vi "Eval y=f(a,x1,x2) Prep.vi"(0 "Variables":string[](array[string]), 1 "formula":string, 2 "Parameters":cluster{string, dbl}[](array[cluster]) {"?" format="%.2f"}, 3 "Start":dbl[](array[numeric]) format="%.2f", 5 "End":dbl[](array[numeric]) format="%.2f") -> (4 "error situation 2":bool, 6 "formula copy":string, 7 "time [msec]":u32, 8 "error situation 1":bool, 9 "error (general)":bool)   [LabVIEW 2017, in "NI_Gmath.lvlib"]
uses:
  NI_Gmath.lvlib
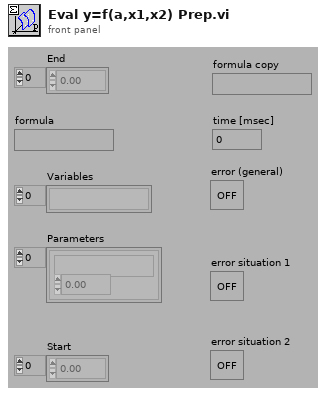
[diagram p1: front panel]
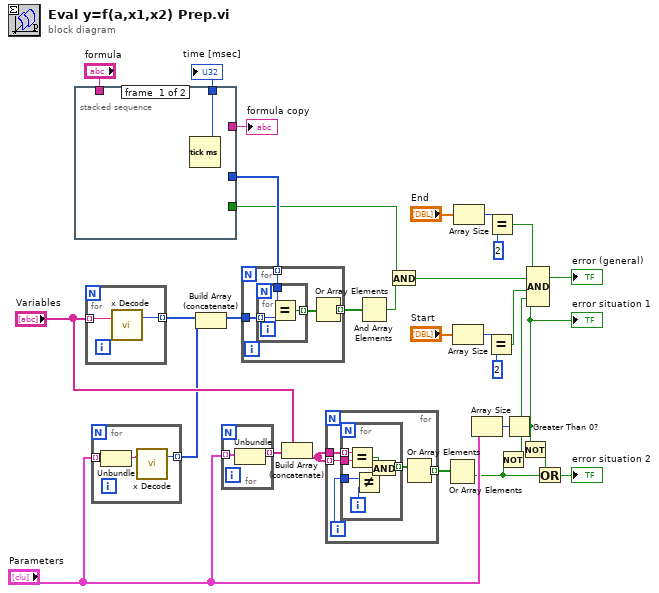
[diagram p0: block diagram]
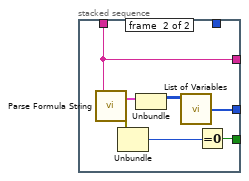
[diagram p2: hidden frame]
diagram:
  n1 = stacked-sequence {
    tunnel: [_ w39] -> w2
    tunnel: [w32 _] -> w4
    tunnel: [_ w38] -> w16
    tunnel: [_ w37] -> w3
    tunnel: "formula" -> [_ w37]
    frame #0 {
      n2 = Tick Count (ms)() -> (millisecond timer value=w32:u32)
    }
    frame #1 {
      n3 = call "Parse Formula String.vi"("formula"=w37) -> ("error out"=w36:errorcluster, "Parsed Formula"=w34:cluster{"Table":i32[][], "Y Values":dbl[]})  [unwired: 1 in]
      n4 = Unbundle(w36) -> ("code"=w35:i32)  [unwired: 2 out]
      n5 = Unbundle(w34) -> ("Table"=w33:i32[][])  [unwired: 1 out]
      n6 = call "List of Variables.vi"("Table"=w33) -> ("List of variables"=w38:i32[])
      n7 = Equal To 0?(x=w35) -> (x = 0?=w39:bool)
    }
  }
  "time [msec]" <- w4
  "formula copy" <- w3
  n8 = for {
    tunnel: "Variables" -> [w41] mode=indexing
    tunnel: [w40] -> w18 mode=indexing
    n9 = call "x Decode.vi"("x string"=w41) -> ("number"=w40:i32)  [unwired: 1 in, 1 out]
  }
  n10 = for {
    tunnel: "Parameters" -> [w43] mode=indexing
    tunnel: [w44] -> w19 mode=indexing
    n11 = Unbundle(w43) -> (w42:string)  [unwired: 1 out]
    n12 = call "x Decode.vi"("x string"=w42) -> ("number"=w44:i32)  [unwired: 1 in, 1 out]
  }
  n13 = Build Array (concatenate)(w18, w19) -> (w20:i32[])
  n14 = for {
    tunnel: "Parameters" -> [w46] mode=indexing
    tunnel: [w45] -> w26 mode=indexing
    n15 = Unbundle(w46) -> (w45:string)  [unwired: 1 out]
  }
  n16 = for {
    tunnel: [w49] -> w17 mode=indexing
    tunnel: w16 -> [w48] mode=indexing
    tunnel: w20 -> [w47]
    n17 = for {
      tunnel: [w53] -> w50 mode=indexing
      tunnel: w48 -> [w52]
      tunnel: w47 -> [w51] mode=indexing
      n18 = Equal?(x=w52, y=w51) -> (x = y?=w53:bool)
    }
    n19 = Or Array Elements(Boolean array=w50) -> (logical OR=w49:bool)
  }
  n20 = Build Array (concatenate)("Variables", w26) -> (w27:string[])
  n21 = for {
    tunnel: w27 -> [w58]
    tunnel: w27 -> [w57] mode=indexing
    tunnel: [w54] -> w21 mode=indexing
    i -> [w56]
    n22 = for {
      tunnel: w58 -> [w65] mode=indexing
      tunnel: w57 -> [w64]
      tunnel: w56 -> [w63]
      tunnel: [w59] -> w55 mode=indexing
      i -> [w62]
      n23 = Equal?(x=w65, y=w64) -> (x = y?=w61:bool)
      n24 = Not Equal?(x=w63, y=w62) -> (x != y?=w60:bool)
      n25 = And(x=w61, y=w60) -> (x .and. y?=w59:bool)
    }
    n26 = Or Array Elements(Boolean array=w55) -> (logical OR=w54:bool)
  }
  n27 = And Array Elements(Boolean array=w17) -> (logical AND=w1:bool)
  n28 = And(x=w2, y=w1) -> (x .and. y?=w12:bool)
  n29 = Or Array Elements(Boolean array=w21) -> (logical OR=w29:bool)
  n30 = Array Size(array="Start") -> (size(s)=w9:i32)
  n31 = Array Size(array="End") -> (size(s)=w6:i32)
  n32 = Array Size(array="Parameters") -> (size(s)=w23:i32)
  n33 = Equal?(x=w9, y=2) -> (x = y?=w15:bool)
  n34 = Equal?(x=w6, y=2) -> (x = y?=w11:bool)
  n35 = Not(x=w29) -> (.not. x?=w22:bool)
  n36 = Greater Than 0?(x=w23) -> (x > 0?=w24:bool)
  "error situation 1" <- w24
  n37 = Not(x=w24) -> (.not. x?=w28:bool)
  n38 = Compound Arithmetic op=AND(w11, w12, w15, w22, w24) -> (→"error (general)":bool)
  n39 = Or(x=w28, y=w29) -> (x .or. y?=→"error situation 2":bool)
